vi "Data Lookup Table.vi"(4 "J1939 Process Parameters":T2={"J1939 XNET Settings"={"XNET Database"="", "XNET Cluster"="", "CAN Port"="", "Baud rate [Bd]"=0, "Termination"=0, "Incoming Rate"=0, "Outcoming Rate"=1, "Write Decimation"=1}, "Incoming Single Point Configuraiton"={"Incoming Single Point Frame"={"ID"=[], "Conversion"=[], "Channel Array Positions"=[], "Frame Length"=[]}, "Channel Pairs"={"Chan Refs"=[], "Previous Chan Values"=[]}, "Read FIFO"=refnum}, "Outgoing Cyclic Configuraiton"={"Outgoing Cyclic Frame"={"ID"=[], "Conversion"=[], "Channel Array Positions"=[], "Frame Length"=[], "Transmit Propreties"=[]}, "Channel Pairs"={"Block Data Refs"=[], "Previous Chan Values"=[]}, "Write FIFO"=refnum}, "J1939 Monitor Settings"={"J1939 Network Address"=0, "Name"=0}, "Simulated Addresses"=[], "Simulated Addresses LUT"=variant} {"Simulated Addresses"."Simulated Addresses"."J1939 XNET Settings"."Name" format="%.0x"; "Simulated Addresses"."Simulated Addresses"."DM1 Data"."Data Reference" format="%.0x"; "Simulated Addresses"."Simulated Addresses"."DM1 Enable?"."Data Reference" format="%.0x"; "Simulated Addresses"."Simulated Addresses"."DM2 Data"."Data Reference" format="%.0x"; "Simulated Addresses"."Simulated Addresses"."DM2 Enable?"."Data Reference" format="%.0x"; "J1939 Monitor Settings"."Name" format="%.0x"; "Outgoing Cyclic Configuraiton"."Channel Pairs"."Block Data Refs"."Data Reference" format="%.0x"; "Outgoing Cyclic Configuraiton"."Outgoing Cyclic Frame"."Transmit Propreties"."Transmit Time" format="%#_p"; "J1939 XNET Settings"."Termination" items=["Off", "On"]; "Incoming Single Point Configuraiton"."Channel Pairs"."Chan Refs" format="%.0x"}, 6 "command":T17, 7 "Direct Access":cluster{"Offset":u32, "Length":u32}, 8 "error in (no error)":errorcluster {"code" min=0 max=0}, 9 "Signals":dbl[](array[numeric]), 10 "ID":u32, 11 "Data Ref":T1) -> (0 "error out":errorcluster {"code" min=0 max=0}, 1 "Signals Out":dbl[](array[numeric]), 3 "Data Ref out":T1)   [LabVIEW 2013, in "J1939 Addon Engine.lvlib"]
uses:
  J1939 Addon Engine.lvlib
  Types/Data Lookup Table Action.ctl
  Types/Process Parameters.ctl
  Shared/Types/XNET Settings.ctl
  Types/Incoming Single Point Configuration.ctl
  Types/Incoming Single Point Frame Pairs.ctl
  Types/Incoming Single Point Channel Pairs.ctl
  <vilib>/NI Veristand/Custom Device API/Data Reference.ctl
  Types/Outgoing Cyclic Configuration.ctl
  Types/Outgoing Cyclic Frame Pairs.ctl
  Shared/Types/XNET Frame Event Properties.ctl
  Types/Outgoing Cyclic Channel Pairs.ctl
  <vilib>/NI Veristand/Custom Device API/Block Data Reference.ctl
  Shared/Types/Monitor Settings.ctl
  Types/Simulated Settings.ctl
  Shared/Types/Compiled Simulated Settings.ctl
  Types/DTC FIFOs.ctl
  Types/Data Lookup Table Reference.ctl
  Types/Datatable Lookup DVR.ctl
  Shared/J1939 Utilities/SubVIs/Convert CAN Arb ID to J1939 ID.vi
  Shared/J1939 Utilities/J1939 Utilities.lvlib
  <vilib>/NI Veristand/Custom Device API/Custom Device API.lvlib
  Shared/J1939 Addon Shared.lvlib
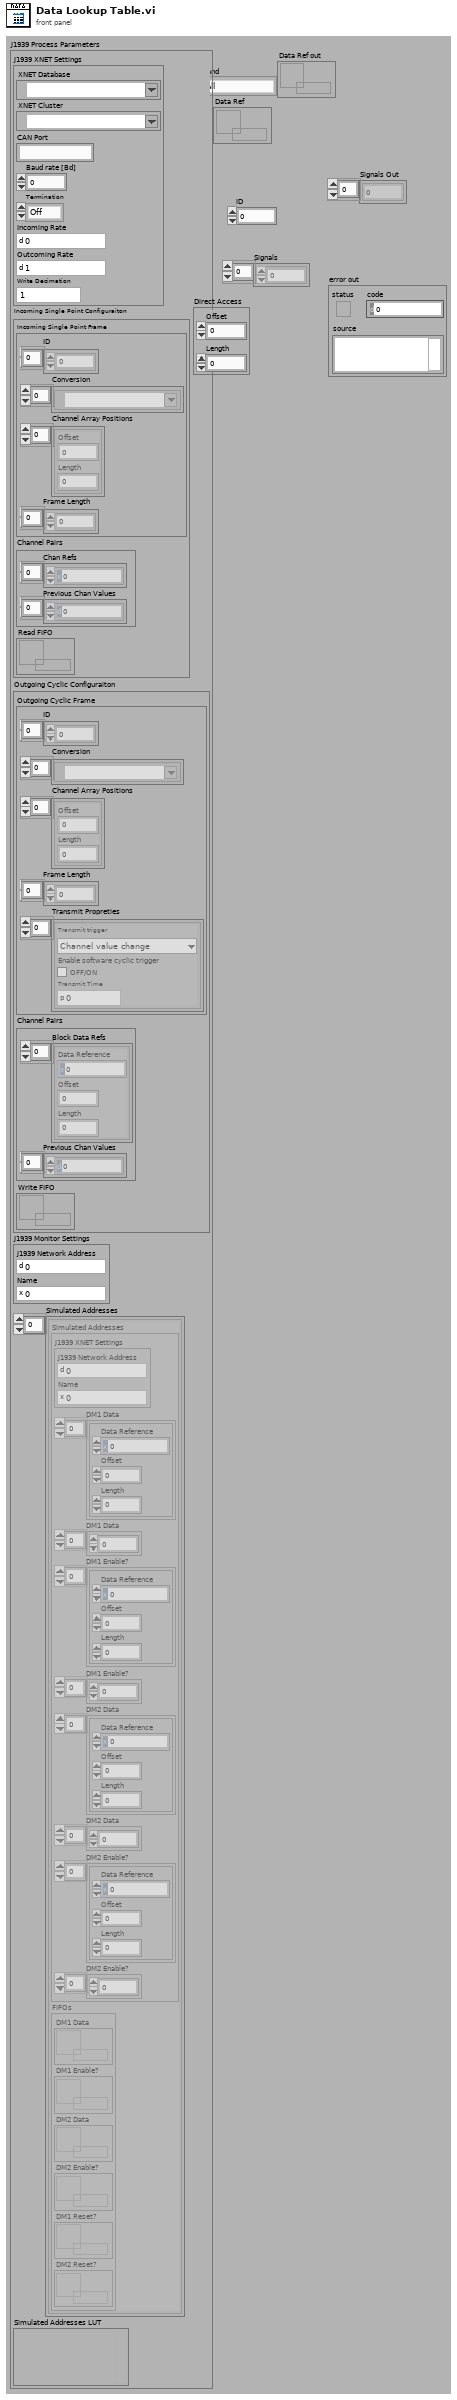
[diagram p1: front panel]
types:
  T1 = typedef "J1939 Addon Engine.lvlib/Data Lookup Table Reference.ctl" = refnum<data-value>
  T2 = typedef "J1939 Addon Engine.lvlib/Process Parameters.ctl" = cluster{"J1939 XNET Settings":T3, "Incoming Single Point Configuraiton":T4, "Outgoing Cyclic Configuraiton":T8, "J1939 Monitor Settings":T13, "Simulated Addresses":T14[], "Simulated Addresses LUT":variant}
  T3 = typedef "J1939 Addon Shared.lvlib/XNET Settings.ctl" = cluster{"XNET Database":refnum<k21>, "XNET Cluster":refnum<k21>, "CAN Port":string, "Baud rate [Bd]":u32, "Termination":u32, "Incoming Rate":u32, "Outcoming Rate":u32, "Write Decimation":u32}
  T4 = typedef "J1939 Addon Engine.lvlib/Incoming Single Point Configuration.ctl" = cluster{"Incoming Single Point Frame":T5, "Channel Pairs":T6, "Read FIFO":refnum<k33>}
  T5 = typedef "J1939 Addon Engine.lvlib/Incoming Single Point Frame Pairs.ctl" = cluster{"ID":u32[], "Conversion":refnum<k21>[], "Channel Array Positions":cluster{"Offset":u32, "Length":u32}[], "Frame Length":u32[]}
  T6 = typedef "J1939 Addon Engine.lvlib/Incoming Single Point Channel Pairs.ctl" = cluster{"Chan Refs":T7[], "Previous Chan Values":dbl[]}
  T7 = typedef "Custom Device API.lvlib/Data Reference.ctl" = i32
  T8 = typedef "J1939 Addon Engine.lvlib/Outgoing Cyclic Configuration.ctl" = cluster{"Outgoing Cyclic Frame":T9, "Channel Pairs":T11, "Write FIFO":refnum<k33>}
  T9 = typedef "J1939 Addon Engine.lvlib/Outgoing Cyclic Frame Pairs.ctl" = cluster{"ID":u32[], "Conversion":refnum<k21>[], "Channel Array Positions":cluster{"Offset":u32, "Length":u32}[], "Frame Length":u32[], "Transmit Propreties":T10[]}
  T10 = typedef "J1939 Addon Shared.lvlib/XNET Frame Event Properties.ctl" = cluster{"Transmit trigger":enum16{"Channel value change"}, "Enable software cyclic trigger":bool, "Transmit Time":dbl}
  T11 = typedef "J1939 Addon Engine.lvlib/Outgoing Cyclic Channel Pairs.ctl" = cluster{"Block Data Refs":T12[], "Previous Chan Values":dbl[]}
  T12 = typedef "Custom Device API.lvlib/Block Data Reference.ctl" = cluster{"Data Reference":T7, "Offset":i32, "Length":i32}
  T13 = typedef "J1939 Addon Shared.lvlib/Monitor Settings.ctl" = cluster{"J1939 Network Address":u8, "Name":u64}
  T14 = typedef "J1939 Addon Engine.lvlib/Simulated Settings.ctl" = cluster{"Simulated Addresses":T15, "FIFOs":T16}
  T15 = typedef "J1939 Addon Shared.lvlib/Compiled Simulated Settings.ctl" = cluster{"J1939 XNET Settings":T13, "DM1 Data":T12[], "DM1 Data":dbl[], "DM1 Enable?":T12[], "DM1 Enable?":dbl[], "DM2 Data":T12[], "DM2 Data":dbl[], "DM2 Enable?":T12[], "DM2 Enable?":dbl[]}
  T16 = typedef "J1939 Addon Engine.lvlib/DTC FIFOs.ctl" = cluster{"DM1 Data":refnum<k33>, "DM1 Enable?":refnum<k33>, "DM2 Data":refnum<k33>, "DM2 Enable?":refnum<k33>, "DM1 Reset?":refnum<k33>, "DM2 Reset?":refnum<k33>}
  T17 = typedef "J1939 Addon Engine.lvlib/Data Lookup Table Action.ctl" = enum16{"Get All", "Set All", "Set Frame", "Get Frame", "Set Range", "Get Range"}
  T18 = typedef "J1939 Addon Engine.lvlib/Datatable Lookup DVR.ctl" = cluster{"LUT":variant, "Signals":dbl[]}
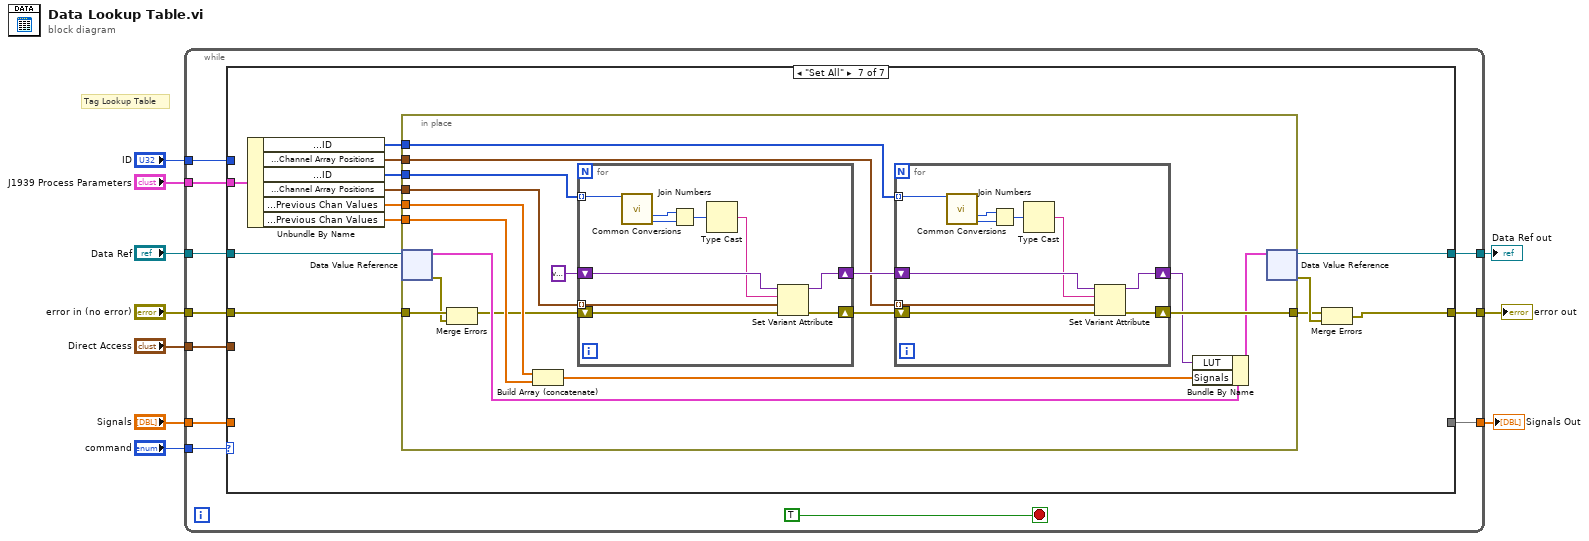
[diagram p0: block diagram]
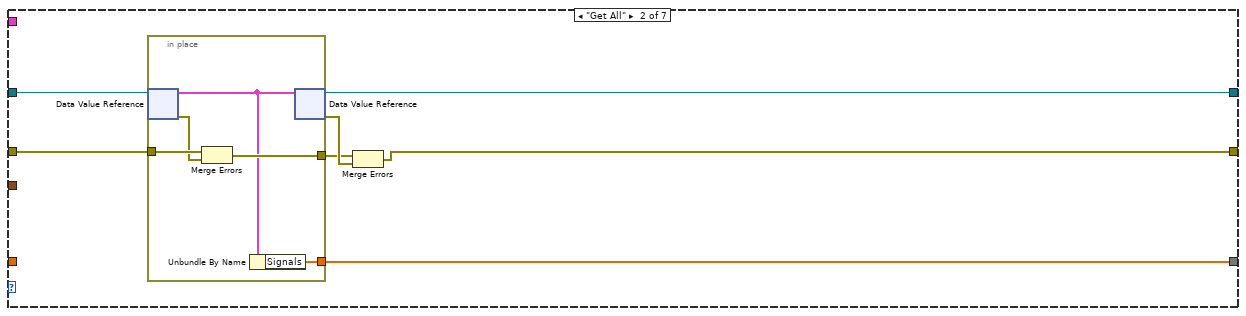
[diagram p3: hidden frame]
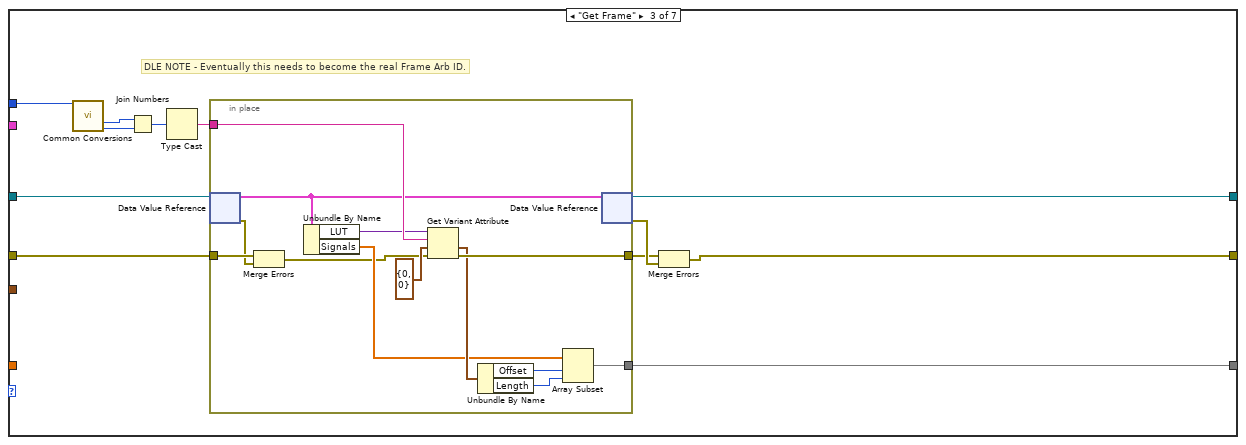
[diagram p4: hidden frame]
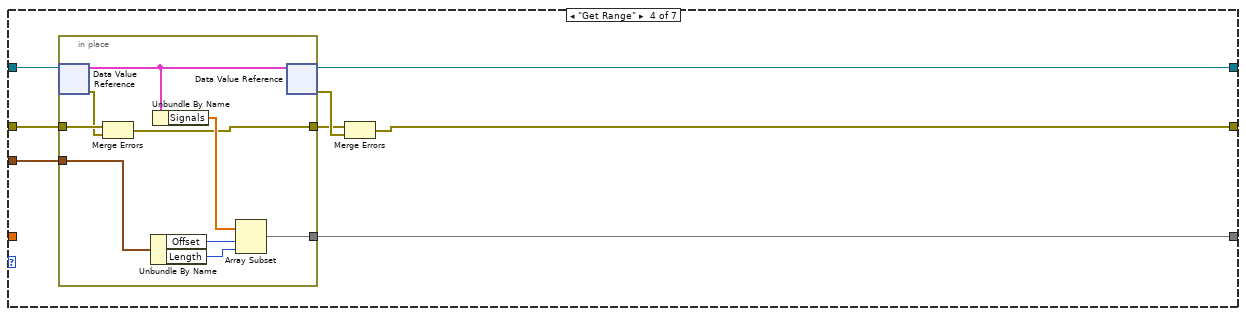
[diagram p5: hidden frame]
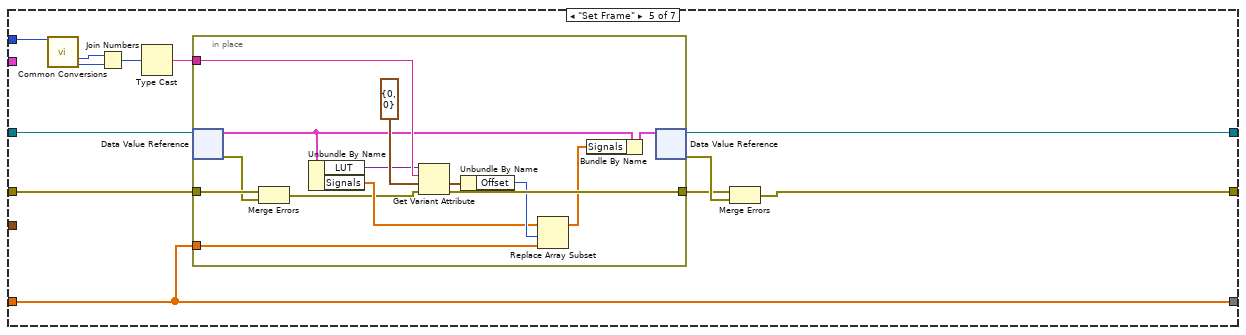
[diagram p6: hidden frame]
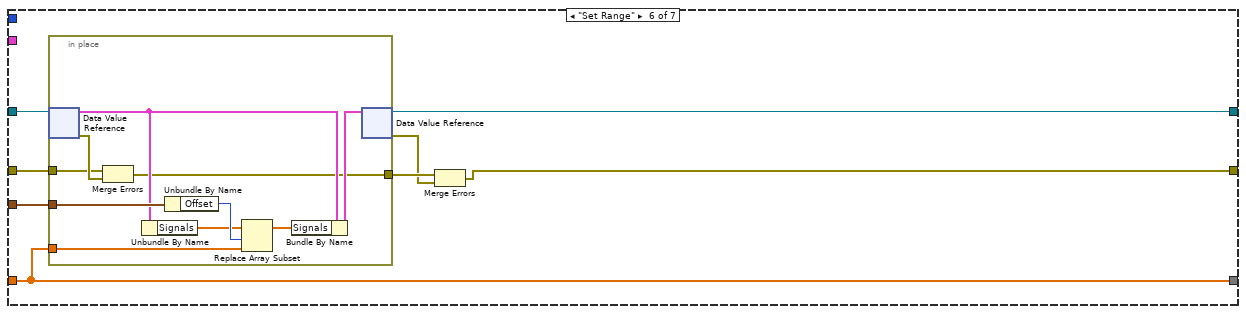
[diagram p7: hidden frame]
diagram:
  # "Tag Lookup Table"
  n1 = while {
    tunnel: "command" -> [w20]
    tunnel: "error in (no error)" -> [w19]
    tunnel: [w18] -> w8
    tunnel: "ID" -> [w17]
    tunnel: "J1939 Process Parameters" -> [w16]
    tunnel: [w15] -> w4
    tunnel: "Signals" -> [w14]
    tunnel: "Direct Access" -> [w13]
    tunnel: "Data Ref" -> [w12]
    tunnel: [w11] -> w1
    stop <- TRUE stop-if-true
    n2 = case shown="\"Set All\"" w20 {
      tunnel: w19 -> [w23 w28 w47 w65 w89 w108 w134]
      tunnel: [w23 w25 w37 w62 w80 w104 w124] -> w18
      tunnel: w17 -> [_ _ w44 _ w86 _ _]
      tunnel: w16 -> [_ _ _ _ _ _ w132]
      tunnel: [_ w29 w45 w66 w87 w111 _] -> w15
      tunnel: w14 -> [_ _ _ _ w87 w111 _]
      tunnel: w13 -> [_ _ _ w67 _ w110 _]
      tunnel: w12 -> [w22 w30 w40 w68 w82 w109 w126]
      tunnel: [w22 w24 w39 w64 w78 w105 w122] -> w11
      frame Default {
      }
      frame "Get All" {
        n3 = in-place {
          in-place-border: [w35] -> w29
          in-place-border: w28 -> [w34]
          in-place-border: [w32] -> w26
          n4 = in-place-dvr #1(w30) -> (w31:T18, w33:errorcluster)
          n5 = Merge Errors(w34, w33) -> (w32:errorcluster)
          n6 = Unbundle By Name(w31) -> ("Signals"=w35:dbl[])
          n7 = in-place-dvr #1(w31) -> (w24:T1, w27:errorcluster)
        }
        n8 = Merge Errors(w26, w27) -> (w25:errorcluster)
      }
      frame "Get Frame" {
        # "DLE NOTE - Eventually this needs to become the real Frame Arb ID."
        n9 = call-poly "Common Conversions.vi"("Arb ID"=w44) -> ("PGN"=w42:u32, "Source Address"=w43:u8)  [unwired: 13 out]
        n10 = Join Numbers(hi=w42, lo=w43) -> ((hi.lo)=w41:u64)
        n11 = Type Cast(x=w41) -> (*(type *) &x=w46:string)  [unwired: 1 in]
        n12 = in-place {
          in-place-border: w47 -> [w60]
          in-place-border: w46 -> [w59]
          in-place-border: [w58] -> w36
          in-place-border: [w53] -> w45
          n13 = in-place-dvr #2(w40) -> (w50:T18, w48:errorcluster)
          n14 = Merge Errors(w60, w48) -> (w49:errorcluster)
          n15 = Unbundle By Name(w50) -> ("LUT"=w52:variant, "Signals"=w51:dbl[])
          n16 = Get Variant Attribute(Variant=w52, name=w59, default value (empty Variant)=cluster{"Offset":u32, "Length":u32} {"Offset"=0, "Length"=0} ("Channel Array Position"), error in=w49) -> (value=w56:cluster{"Offset":u32, "Length":u32}, error out=w58:errorcluster)  [unwired: 2 out]
          n17 = Unbundle By Name(w56) -> ("Offset"=w54:u32, "Length"=w55:u32)
          n18 = Array Subset(array=w51, index=w54, length=w55) -> (w53:dbl[])
          n19 = in-place-dvr #2(w50) -> (w39:T1, w38:errorcluster)
        }
        n20 = Merge Errors(w36, w38) -> (w37:errorcluster)
      }
      frame "Get Range" {
        n21 = in-place {
          in-place-border: w65 -> [w77]
          in-place-border: [w69] -> w61
          in-place-border: [w74] -> w66
          in-place-border: w67 -> [w70]
          n22 = in-place-dvr #3(w68) -> (w72:T18, w71:errorcluster)
          n23 = Merge Errors(w77, w71) -> (w69:errorcluster)
          n24 = Unbundle By Name(w70) -> ("Offset"=w75:u32, "Length"=w76:u32)
          n25 = Unbundle By Name(w72) -> ("Signals"=w73:dbl[])
          n26 = Array Subset(array=w73, index=w75, length=w76) -> (w74:dbl[])
          n27 = in-place-dvr #3(w72) -> (w64:T1, w63:errorcluster)
        }
        n28 = Merge Errors(w61, w63) -> (w62:errorcluster)
      }
      frame "Set Frame" {
        n29 = call-poly "Common Conversions.vi"("Arb ID"=w86) -> ("PGN"=w84:u32, "Source Address"=w85:u8)  [unwired: 13 out]
        n30 = Join Numbers(hi=w84, lo=w85) -> ((hi.lo)=w83:u64)
        n31 = Type Cast(x=w83) -> (*(type *) &x=w88:string)  [unwired: 1 in]
        n32 = in-place {
          in-place-border: w89 -> [w103]
          in-place-border: w88 -> [w102]
          in-place-border: [w101] -> w79
          in-place-border: w87 -> [w97]
          n33 = in-place-dvr #4(w82) -> (w96:T18, w90:errorcluster)
          n34 = Merge Errors(w103, w90) -> (w91:errorcluster)
          n35 = Unbundle By Name(w96) -> ("LUT"=w92:variant, "Signals"=w93:dbl[])
          n36 = Get Variant Attribute(Variant=w92, name=w102, default value (empty Variant)=cluster{"Offset":u32, "Length":u32} {"Offset"=0, "Length"=0} ("Channel Array Position"), error in=w91) -> (value=w99:cluster{"Offset":u32, "Length":u32}, error out=w101:errorcluster)  [unwired: 2 out]
          n37 = Unbundle By Name(w99) -> ("Offset"=w98:u32)
          n38 = Replace Array Subset(array=w93, new element=w97, index=w98) -> (w95:dbl[])
          n39 = Bundle By Name(cluster=w96, "Signals"=w95) -> (w94:T18)
          n40 = in-place-dvr #4(w94) -> (w78:T1, w81:errorcluster)
        }
        n41 = Merge Errors(w79, w81) -> (w80:errorcluster)
      }
      frame "Set Range" {
        n42 = in-place {
          in-place-border: w111 -> [w120]
          in-place-border: w110 -> [w119]
          in-place-border: w108 -> [w113]
          in-place-border: [w112] -> w107
          n43 = in-place-dvr #5(w109) -> (w117:T18, w114:errorcluster)
          n44 = Merge Errors(w113, w114) -> (w112:errorcluster)
          n45 = Unbundle By Name(w117) -> ("Signals"=w118:dbl[])
          n46 = Unbundle By Name(w119) -> ("Offset"=w121:u32)
          n47 = Replace Array Subset(array=w118, new element=w120, index=w121) -> (w116:dbl[])
          n48 = Bundle By Name(cluster=w117, "Signals"=w116) -> (w115:T18)
          n49 = in-place-dvr #5(w115) -> (w105:T1, w106:errorcluster)
        }
        n50 = Merge Errors(w107, w106) -> (w104:errorcluster)
      }
      frame "Set All" {
        n51 = Unbundle By Name(w132) -> ("Outgoing Cyclic Configuraiton.Outgoing Cyclic Frame.ID"=w130:u32[], "Outgoing Cyclic Configuraiton.Outgoing Cyclic Frame.Channel Array Positions"=w129:cluster{"Offset":u32, "Length":u32}[], "Incoming Single Point Configuraiton.Incoming Single Point Frame.ID"=w133:u32[], "Incoming Single Point Configuraiton.Incoming Single Point Frame.Channel Array Positions"=w131:cluster{"Offset":u32, "Length":u32}[], "Incoming Single Point Configuraiton.Channel Pairs.Previous Chan Values"=w127:dbl[], "Outgoing Cyclic Configuraiton.Channel Pairs.Previous Chan Values"=w128:dbl[])
        n52 = in-place {
          in-place-border: w134 -> [w137]
          in-place-border: w133 -> [w150]
          in-place-border: w131 -> [w149]
          in-place-border: [w146] -> w123
          in-place-border: w130 -> [w145]
          in-place-border: w129 -> [w144]
          in-place-border: w128 -> [w143]
          in-place-border: w127 -> [w142]
          n53 = in-place-dvr #6(w126) -> (w141:T18, w136:errorcluster)
          n54 = Merge Errors(w137, w136) -> (w135:errorcluster)
          n55 = Build Array (concatenate)(w142, w143) -> (w140:dbl[])
          n56 = for {
            shift-right: [w170] -> w147
            shift-left: variant ("variant") -> [w171]
            shift-right: [w168] -> w148
            shift-left: w135 -> [w169]
            tunnel: w150 -> [w165] mode=indexing
            tunnel: w149 -> [w166] mode=indexing
            n57 = call-poly "Common Conversions.vi"("Arb ID"=w165) -> ("PGN"=w164:u32, "Source Address"=w162:u8)  [unwired: 13 out]
            n58 = Join Numbers(hi=w164, lo=w162) -> ((hi.lo)=w163:u64)
            n59 = Type Cast(x=w163) -> (*(type *) &x=w167:string)  [unwired: 1 in]
            n60 = Set Variant Attribute(Variant=w171, name=w167, value=w166, error in=w169) -> (Variant out=w170:variant, error out=w168:errorcluster)  [unwired: 1 out]
          }
          n61 = for {
            shift-right: [w160] -> w139
            shift-left: w147 -> [w161]
            shift-right: [w158] -> w146
            shift-left: w148 -> [w159]
            tunnel: w145 -> [w155] mode=indexing
            tunnel: w144 -> [w156] mode=indexing
            n62 = call-poly "Common Conversions.vi"("Arb ID"=w155) -> ("PGN"=w154:u32, "Source Address"=w153:u8)  [unwired: 13 out]
            n63 = Join Numbers(hi=w154, lo=w153) -> ((hi.lo)=w152:u64)
            n64 = Type Cast(x=w152) -> (*(type *) &x=w157:string)  [unwired: 1 in]
            n65 = Set Variant Attribute(Variant=w161, name=w157, value=w156, error in=w159) -> (Variant out=w160:variant, error out=w158:errorcluster)  [unwired: 1 out]
          }
          n66 = Bundle By Name(cluster=w141, "LUT"=w139, "Signals"=w140) -> (w138:T18)
          n67 = in-place-dvr #6(w138) -> (w122:T1, w125:errorcluster)
        }
        n68 = Merge Errors(w123, w125) -> (w124:errorcluster)
      }
    }
  }
  "error out" <- w8
  "Signals Out" <- w4
  "Data Ref out" <- w1
